vi "Begin.vi"() -> (0 "error out":errorcluster)   [LabVIEW 2013]
doc: "Called before other user functions, this VI is expected to open initial I/O refnums, load in file data, and do all program initialization. Notice that the <B>error out</B> terminal is simply used for data flow. Wiring it to other structures or subVIs ensures that this VI runs first."
uses:
  <vilib>/Rock Robotics/WPI/SafetyOutput/WPI_SafetyOutputConfigMenu.ctl
  <vilib>/Rock Robotics/WPI/DriverStation/WPI_DriverStationRobotMode2.ctl
  <vilib>/Rock Robotics/WPI/Joystick/WPI_JoystickDeviceEnum.ctl
  <vilib>/Rock Robotics/SystemInterfaces/DIO/FPGA_DIORelayChannel.ctl
  <vilib>/Rock Robotics/SystemInterfaces/DIO/FPGA_DIOChannel.ctl
  <vilib>/Rock Robotics/SystemInterfaces/Typedef/FPGA_TypedefDigitalModule.ctl
  <vilib>/Rock Robotics/WPI/Solenoid/WPI_SolenoidChannel.ctl
  TankDriveAction.ctl
  QueueAction.ctl
  <vilib>/Rock Robotics/SystemInterfaces/Typedef/FPGA_TypedefSolenoidModule.ctl
  DoubleSolenoidAction.ctl
  RollerAction.ctl
  CollectorAction.ctl
  <vilib>/Rock Robotics/SystemInterfaces/DIO/FPGA_DIOPWMChannel.ctl
  SonarAction.ctl
  <vilib>/Rock Robotics/SystemInterfaces/AI/FPGA_AIChannel.ctl
  <vilib>/Rock Robotics/SystemInterfaces/Typedef/FPGA_TypedefAnalogModule.ctl
  PressureSensorAction.ctl
  Robot Global Data.vi
  OutputErrors.vi
  <vilib>/Rock Robotics/WPI/Solenoid/WPI_SolenoidOpenSingle.vi
  <vilib>/Rock Robotics/WPI/MotorControl/WPI_MotorControlOpen Talon.vi
  <vilib>/Rock Robotics/WPI/RobotDrive/WPI_RobotDriveOpen4MotorWithTalon.vi
  <vilib>/Rock Robotics/WPI/Compressor/WPI_CompressorGetSetRefNum.vi
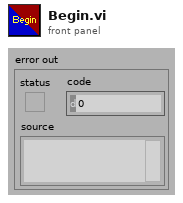
[diagram p1: front panel]
types:
  T1 = typedef "FPGA_DIOPWMChannel.ctl" = enum8{"PWM 1", "PWM 2", "PWM 3", "PWM 4", "PWM 5", "PWM 6", "PWM 7", "PWM 8", "PWM 9", "PWM 10", "Invalid"}
  T2 = typedef "PressureSensorAction.ctl" = enum16{"Init", "ReadValue", "Disable"}
  T3 = typedef "FPGA_AIChannel.ctl" = enum8{"AI 1", "AI 2", "AI 3", "AI 4", "AI 5", "AI 6", "AI 7", "AI 8", "Invalid"}
  T4 = typedef "FPGA_TypedefAnalogModule.ctl" = enum16{"Analog Module 1", "Analog Module 2"}
  T5 = typedef "SonarAction.ctl" = enum16{"Init", "ReadValue", "Disable"}
  T6 = typedef "FPGA_DIOChannel.ctl" = enum8{"DIO 1", "DIO 2", "DIO 3", "DIO 4", "DIO 5", "DIO 6", "DIO 7", "DIO 8", "DIO 9", "DIO 10", "DIO 11", "DIO 12", "DIO 13", "DIO 14", "Invalid"}
  T7 = typedef "CollectorAction.ctl" = enum16{"Init", "Raise", "Lower", "Stop", "GetStatus"}
  T8 = typedef "RollerAction.ctl" = enum16{"Init", "Off", "Forward", "Reverse"}
  T9 = typedef "FPGA_DIORelayChannel.ctl" = enum8{"Relay 1", "Relay 2", "Relay 3", "Relay 4", "Relay 5", "Relay 6", "Relay 7", "Relay 8", "Invalid"}
  T10 = typedef "FPGA_TypedefDigitalModule.ctl" = enum16{"Digital Module 1", "Digital Module 2"}
  T11 = typedef "DoubleSolenoidAction.ctl" = enum16{"Init", "Middle", "In", "Out"}
  T12 = typedef "WPI_SolenoidChannel.ctl" = enum8{"Solenoid 1", "Solenoid 2", "Solenoid 3", "Solenoid 4", "Solenoid 5", "Solenoid 6", "Solenoid 7", "Solenoid 8", "Invalid"}
  T13 = typedef "FPGA_TypedefSolenoidModule.ctl" = enum16{"Solenoid Module 1", "Solenoid Module 2"}
  T14 = typedef "QueueAction.ctl" = enum16{"Init", "SetValue", "Disable"}
  T15 = typedef "TankDriveAction.ctl" = enum16{"Init", "LinearDrive", "SetValue", "Disable"}
  T16 = typedef "WPI_JoystickDeviceEnum.ctl" = enum16{"USB 1", "USB 2", "USB 3", "USB 4", "Kinect 1", "Kinect 2"}
  T17 = typedef "WPI_DriverStationRobotMode2.ctl" = enum16{"Autonomous Disabled", "Autonomous Enabled", "Teleop Disabled", "Teleop Enabled", "Timeout", "Finish", "Test Disabled", "Test Enabled"}
  T18 = typedef "WPI_SafetyOutputConfigMenu.ctl" = enum16{"Enable", "Disable"}
  T19 = typedef "WPI_JoystickDevRef.ctl" = cluster{"Device":T16}
  T20 = typedef "WPI_RobotDriveDevRef.ctl" = cluster{"DevStatus":errorcluster, "Motors[]":T21[], "Square Inputs":bool, "Max Output":dbl, "Isochronous":bool}
  T21 = typedef "WPI_MotorControlDeviceRef.ctl" = cluster{"DeviceStatus":errorcluster, "Type":enum16{"PWM", "CAN"}, "PWM":cluster{"Digital Module":T10, "PWM Channel":T1, "DeadBand":T22}, "CAN":cluster{"Device Number":u8, "Control Mode":T23, "Semaphore":T24, "Max Vout":dbl}, "Invert":bool, "TransformRef":T25, "InvTransformRef":T25}
  T22 = typedef "WPI_PWMDeadband.ctl" = cluster{"Name":string, "maxPositivePwm":i32, "minPositivePwm":i32, "centerPwm":i32, "maxNegativePwm":i32, "minNegativePwm":i32, "angularRange":u16}
  T23 = typedef "WPI_CANJaguar_ControlMode.ctl" = enum8{"Percent VBus", "Current", "Speed", "Position", "Voltage"}
  T24 = typedef "Semaphore RefNum" = refnum<k1>
  T25 = typedef "WPI_PWMTransform_ConPane.ctl" = refnum<vi>
  T26 = typedef "WPI_CompressorDevRef.ctl" = cluster{"DevStatus":errorcluster, "DigitalInputDevRef":T27, "RelayDevRef":T28}
  T27 = typedef "WPI_DigitalInputDevRef.ctl" = cluster{"DevStatus":errorcluster, "DIO Channel":T6, "Digital Module":T10}
  T28 = typedef "WPI_RelayDevRef.ctl" = cluster{"DevStatus":errorcluster, "Relay Channel":T9, "Digital Module":T10, "Relay Direction":T29}
  T29 = typedef "WPI_RelayDirection.ctl" = enum16{"Both directions", "Forward only", "Reverse only"}
  T30 = typedef "WPI_SolenoidDevRef.ctl" = cluster{"DevStatus":errorcluster, "Solenoid Module":T13, "Forward Solenoid Channel":T12, "Reverse Solenoid Channel":T12}
  T31 = typedef "WPI_AnalogChannelDevRef.ctl" = cluster{"DevStatus":errorcluster, "Analog Module":T4, "Analog Channel":T3}
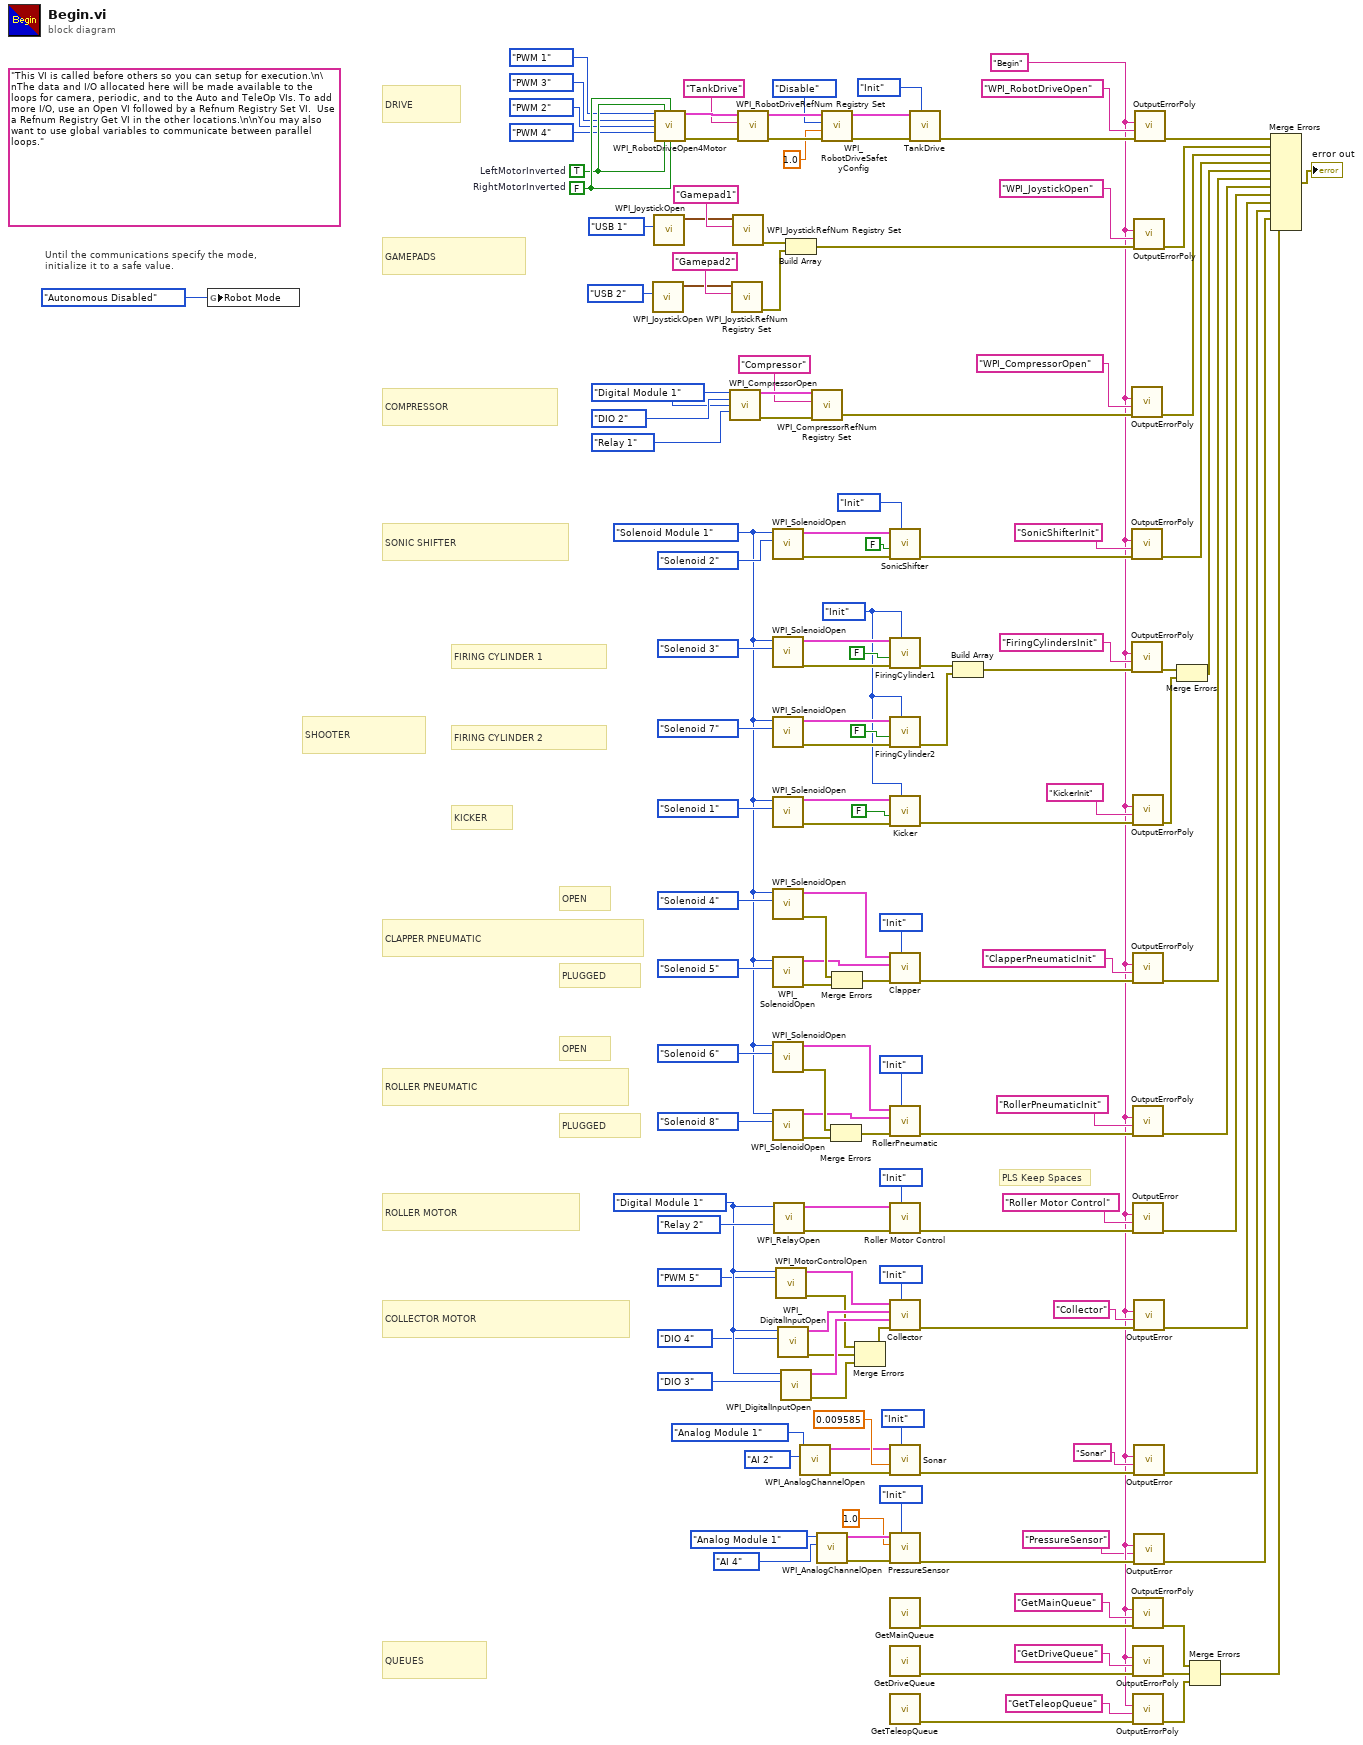
[diagram p0: block diagram]
diagram:
  w34 = FPGA_TypedefDigitalModule."Digital Module 1" ("Digital Module (Module 1)")
  w57 = FPGA_TypedefSolenoidModule."Solenoid Module 1" ("Solenoid Module (Module 1)")
  w80 = QueueAction."Init" ("Action")
  w126 = FPGA_TypedefDigitalModule."Digital Module 1" ("Pressure Switch\nand Relay Module")
  w14 = "Begin"
  (unwired) "This VI is called before others so you can setup for execution.\n\nThe data and I/O allocated here will be made available to the loops for camera, periodic, and to the Auto and TeleOp VIs. To add more I/O, use an Open VI followed by a Refnum Registry Set VI.  Use a Refnum Registry Get VI in the other locations.\n\nYou may also want to use global variables to communicate between parallel loops."
  w5 = TRUE  # LeftMotorInverted
  w6 = FALSE  # RightMotorInverted
  # "COLLECTOR MOTOR"
  # "PLS Keep Spaces"
  # "ROLLER MOTOR"
  # "PLUGGED"
  # "OPEN"
  # "PLUGGED"
  # "OPEN"
  # "ROLLER PNEUMATIC"
  # "CLAPPER PNEUMATIC"
  # "SONIC SHIFTER"
  # "QUEUES"
  # "KICKER"
  # "FIRING CYLINDER 2"
  # "FIRING CYLINDER 1"
  # "SHOOTER"
  # "COMPRESSOR"
  # "GAMEPADS"
  # "DRIVE"
  # "Until the communications specify the mode,\ninitialize it to a safe value."
  n1 = global write "Robot Global Data.vi" "Robot Mode"(WPI_DriverStationRobotMode2."Autonomous Disabled" ("Robot Mode")) -> ()
  n2 = call <vilib>:"WPI_JoystickOpen.vi"("JoystickDevice"=WPI_JoystickDeviceEnum."USB 2") -> ("JoystickDevRef"=w122:T19)  [unwired: 10 in]
  n3 = call <vilib>:"WPI_JoystickOpen.vi"("JoystickDevice"=WPI_JoystickDeviceEnum."USB 1") -> ("JoystickDevRef"=w138:T19)  [unwired: 10 in]
  n4 = call-poly <vilib>:"WPI_RobotDriveOpen4Motor.vi"("Rear Left Motor"=FPGA_DIOPWMChannel."PWM 1", "Rear Left Motor Inverted"=w5, "Rear Right Motor Inverted"=w6, "Rear Right Motor"=FPGA_DIOPWMChannel."PWM 3", "Front Left Motor"=FPGA_DIOPWMChannel."PWM 2", "Front Right Motor"=FPGA_DIOPWMChannel."PWM 4", "Front Left Motor Inverted"=w5, "Front Right Motor Inverted"=w6) -> ("RobotDriveDevRef"=w145:T20, "error out"=w143:errorcluster)  [unwired: 6 in]
  n5 = call <vilib>:"WPI_CompressorOpen.vi"("Pressure Switch Digital Module (Module 1)"=w126, "Pressure Switch DIO Channel"=FPGA_DIOChannel."DIO 2" ("Pressure Switch Channel"), "Relay Digital Module (Module 1)"=w126, "Relay Channel"=FPGA_DIORelayChannel."Relay 1") -> ("CompressorDevRef"=w130:T26, "error out"=w128:errorcluster)  [unwired: 1 in, 9 out]
  n6 = call <vilib>:"WPI_JoystickRefNum Registry Set.vi"("refnum name"="Gamepad2", "JoystickDevRef"=w122) -> ("error out"=w119:errorcluster)  [unwired: 8 in, 1 out]
  n7 = call <vilib>:"WPI_JoystickRefNum Registry Set.vi"("refnum name"="Gamepad1", "JoystickDevRef"=w138) -> ("error out"=w120:errorcluster)  [unwired: 8 in, 1 out]
  n8 = call <vilib>:"WPI_RobotDriveRefNum Registry Set.vi"("error in (no error)"=w143, "refnum name"="TankDrive", "RobotDriveDevRef"=w145) -> ("error out"=w136:errorcluster, "RobotDriveDevRef"=w142:T20)  [unwired: 7 out]
  n9 = call-poly <vilib>:"WPI_SolenoidOpen.vi"("Solenoid Channel"=WPI_SolenoidChannel."Solenoid 2", "Solenoid Module (Module 1)"=w57) -> ("error out"=w76:errorcluster, "SolenoidDevRef"=w77:T30)  [unwired: 8 in]
  n10 = call-poly <vilib>:"WPI_SolenoidOpen.vi"("Solenoid Channel"=WPI_SolenoidChannel."Solenoid 3", "Solenoid Module (Module 1)"=w57) -> ("error out"=w107:errorcluster, "SolenoidDevRef"=w110:T30)  [unwired: 8 in]
  n11 = call-poly <vilib>:"WPI_SolenoidOpen.vi"("Solenoid Channel"=WPI_SolenoidChannel."Solenoid 7", "Solenoid Module (Module 1)"=w57) -> ("error out"=w109:errorcluster, "SolenoidDevRef"=w106:T30)  [unwired: 8 in]
  n12 = call-poly <vilib>:"WPI_SolenoidOpen.vi"("Solenoid Channel"=WPI_SolenoidChannel."Solenoid 1", "Solenoid Module (Module 1)"=w57) -> ("error out"=w108:errorcluster, "SolenoidDevRef"=w105:T30)  [unwired: 8 in]
  n13 = call-poly <vilib>:"WPI_SolenoidOpen.vi"("Solenoid Channel"=WPI_SolenoidChannel."Solenoid 4", "Solenoid Module (Module 1)"=w57) -> ("error out"=w69:errorcluster, "SolenoidDevRef"=w67:T30)  [unwired: 8 in]
  n14 = call-poly <vilib>:"WPI_SolenoidOpen.vi"("Solenoid Channel"=WPI_SolenoidChannel."Solenoid 5", "Solenoid Module (Module 1)"=w57) -> ("error out"=w68:errorcluster, "SolenoidDevRef"=w65:T30)  [unwired: 8 in]
  n15 = call-poly <vilib>:"WPI_SolenoidOpen.vi"("Solenoid Channel"=WPI_SolenoidChannel."Solenoid 6", "Solenoid Module (Module 1)"=w57) -> ("error out"=w60:errorcluster, "SolenoidDevRef"=w55:T30)  [unwired: 8 in]
  n16 = call-poly <vilib>:"WPI_SolenoidOpen.vi"("Solenoid Channel"=WPI_SolenoidChannel."Solenoid 8", "Solenoid Module (Module 1)"=w57) -> ("error out"=w59:errorcluster, "SolenoidDevRef"=w54:T30)  [unwired: 8 in]
  n17 = call <vilib>:"WPI_RelayOpen.vi"("Relay Channel"=FPGA_DIORelayChannel."Relay 2", "Digital Module (Module 1)"=w34) -> ("error out"=w45:errorcluster, "RelayDevRef"=w47:T28)  [unwired: 8 in]
  n18 = call-poly <vilib>:"WPI_MotorControlOpen.vi"("PWM Channel"=FPGA_DIOPWMChannel."PWM 5", "Digital Module (Module 1)"=w34) -> ("error out"=w29:errorcluster, "MotorControlDeviceRef"=w40:T21)  [unwired: 8 in]
  n19 = call <vilib>:"WPI_DigitalInputOpen.vi"("DIO Channel"=FPGA_DIOChannel."DIO 4", "Digital Module (Module 1)"=w34) -> ("error out"=w28:errorcluster, "DigitalInputDevRef"=w36:T27)  [unwired: 8 in]
  n20 = call <vilib>:"WPI_DigitalInputOpen.vi"("DIO Channel"=FPGA_DIOChannel."DIO 3", "Digital Module (Module 1)"=w34) -> ("error out"=w27:errorcluster, "DigitalInputDevRef"=w35:T27)  [unwired: 8 in]
  n21 = Build Array(w120, w119) -> (w118:errorcluster[])
  n22 = call <vilib>:"WPI_AnalogChannelOpen.vi"("Analog Channel"=FPGA_AIChannel."AI 2", "Analog Module (Module 1)"=FPGA_TypedefAnalogModule."Analog Module 1") -> ("error out"=w19:errorcluster, "AIDeviceRef"=w18:T31)  [unwired: 8 in]
  n23 = call <vilib>:"WPI_CompressorRefNum Registry Set.vi"("error in (no error)"=w128, "refnum name"="Compressor", "CompressorDevRef"=w130) -> ("error out"=w125:errorcluster)  [unwired: 7 in, 1 out]
  n24 = call <vilib>:"WPI_AnalogChannelOpen.vi"("Analog Channel"=FPGA_AIChannel."AI 4", "Analog Module (Module 1)"=FPGA_TypedefAnalogModule."Analog Module 1") -> ("error out"=w8:errorcluster, "AIDeviceRef"=w9:T31)  [unwired: 8 in]
  n25 = call <vilib>:"WPI_RobotDriveSafetyConfig.vi"("error in (no error)"=w136, "timeout (s)"=1.0, "mode"=WPI_SafetyOutputConfigMenu."Disable", "RobotDriveDevRef"=w142) -> ("error out"=w91:errorcluster, "RobotDriveDevRef"=w92:T20)  [unwired: 6 in]
  n26 = Merge Errors(w60, w59) -> (w56:errorcluster)
  n27 = Merge Errors(w69, w68) -> (w70:errorcluster)
  n28 = Merge Errors(w29, w28, w27) -> (w30:errorcluster)
  n29 = call "SonicShifter.vi"("Action"=QueueAction."Init", "error in (no error)"=w76, "Default Position"=FALSE, "SolenoidDevRef"=w77) -> ("error out"=w74:errorcluster)  [unwired: 7 in]
  n30 = call "FiringCylinder1.vi"("Action"=w80, "error in (no error)"=w107, "Default Position"=FALSE, "SolenoidDevRef"=w110) -> ("error out"=w112:errorcluster)  [unwired: 7 in]
  n31 = call "FiringCylinder2.vi"("Action"=w80, "error in (no error)"=w109, "Default Position"=FALSE, "SolenoidDevRef"=w106) -> ("error out"=w113:errorcluster)  [unwired: 7 in]
  n32 = call "Kicker.vi"("Action"=w80, "error in (no error)"=w108, "Default Position"=FALSE, "SolenoidDevRef"=w105) -> ("error out"=w114:errorcluster)  [unwired: 7 in]
  n33 = call "Clapper.vi"("State"=DoubleSolenoidAction."Init", "Error in"=w70, "Plugged"=w65, "Open"=w67) -> ("Error out"=w63:errorcluster)  [unwired: 7 in]
  n34 = call "RollerPneumatic.vi"("State"=DoubleSolenoidAction."Init", "Error in"=w56, "Plugged"=w54, "Open"=w55) -> ("Error out"=w53:errorcluster)  [unwired: 7 in]
  n35 = call "Roller Motor Control.vi"("Action"=RollerAction."Init", "Error in"=w45, "RelayDevRef"=w47) -> ("Error out"=w44:errorcluster)  [unwired: 8 in]
  n36 = call "Collector.vi"("Action"=CollectorAction."Init", "Error in"=w30, "BottomLS"=w35, "TopLS"=w36, "Motor"=w40) -> ("Error out"=w38:errorcluster)  [unwired: 4 in, 2 out]
  n37 = call "Sonar.vi"("Action"=SonarAction."Init", "error in (no error)"=w19, "Scaling factor (V/in)"=0.009585, "AIDeviceRef"=w18) -> ("error out"=w26:errorcluster)  [unwired: 6 in, 1 out]
  n38 = call "PressureSensor.vi"("Action"=PressureSensorAction."Init", "error in (no error)"=w8, "PressureScaler"=1.0, "AIDeviceRef"=w9) -> ("error out"=w15:errorcluster)  [unwired: 6 in, 1 out]
  n39 = call "GetMainQueue.vi"() -> ("error out"=w89:errorcluster)  [unwired: 10 in, 1 out]
  n40 = call "GetDriveQueue.vi"() -> ("error out"=w88:errorcluster)  [unwired: 10 in, 1 out]
  n41 = call "GetTeleopQueue.vi"() -> ("error out"=w87:errorcluster)  [unwired: 10 in, 1 out]
  n42 = call "TankDrive.vi"("DriveAction"=TankDriveAction."Init", "error in (no error)"=w91, "RobotDriveDevRef"=w92) -> ("error out"=w90:errorcluster)  [unwired: 7 in, 1 out]
  n43 = Build Array(w112, w113) -> (w111:errorcluster[])
  n44 = call-poly "OutputErrorPoly.vi"("error in (no error)"=w125, "Causing VI"="WPI_CompressorOpen" ("Calling VI"), "Calling VI"=w14) -> ("error out"=w115:errorcluster)  [unwired: 8 in]
  n45 = call-poly "OutputErrorPoly.vi"("error in (no error)"=w74, "Causing VI"="SonicShifterInit", "Calling VI"=w14) -> ("error out"=w72:errorcluster)  [unwired: 8 in]
  n46 = call-poly "OutputErrorPoly.vi"("errors in"=w111, "Causing VI"="FiringCylindersInit", "Calling VI"=w14) -> ("error out"=w101:errorcluster)  [unwired: 8 in]
  n47 = call-poly "OutputErrorPoly.vi"("error in (no error)"=w114, "Causing VI"="KickerInit", "Calling VI"=w14) -> ("error out"=w100:errorcluster)  [unwired: 8 in]
  n48 = call-poly "OutputErrorPoly.vi"("error in (no error)"=w63, "Causing VI"="ClapperPneumaticInit", "Calling VI"=w14) -> ("error out"=w50:errorcluster)  [unwired: 8 in]
  n49 = call-poly "OutputErrorPoly.vi"("error in (no error)"=w53, "Causing VI"="RollerPneumaticInit", "Calling VI"=w14) -> ("error out"=w49:errorcluster)  [unwired: 8 in]
  n50 = call "OutputError.vi"("error in (no error)"=w44, "Causing VI"="Roller Motor Control", "Calling VI"=w14) -> ("error out"=w43:errorcluster)  [unwired: 8 in]
  n51 = call-poly "OutputErrorPoly.vi"("error in (no error)"=w89, "Causing VI"="GetMainQueue", "Calling VI"=w14) -> ("error out"=w84:errorcluster)  [unwired: 8 in]
  n52 = call-poly "OutputErrorPoly.vi"("error in (no error)"=w88, "Causing VI"="GetDriveQueue", "Calling VI"=w14) -> ("error out"=w85:errorcluster)  [unwired: 8 in]
  n53 = call-poly "OutputErrorPoly.vi"("error in (no error)"=w87, "Causing VI"="GetTeleopQueue", "Calling VI"=w14) -> ("error out"=w86:errorcluster)  [unwired: 8 in]
  n54 = call-poly "OutputErrorPoly.vi"("errors in"=w118, "Causing VI"="WPI_JoystickOpen", "Calling VI"=w14) -> ("error out"=w117:errorcluster)  [unwired: 8 in]
  n55 = call "OutputError.vi"("error in (no error)"=w38, "Causing VI"="Collector", "Calling VI"=w14) -> ("error out"=w37:errorcluster)  [unwired: 8 in]
  n56 = call "OutputError.vi"("error in (no error)"=w26, "Causing VI"="Sonar", "Calling VI"=w14) -> ("error out"=w23:errorcluster)  [unwired: 8 in]
  n57 = call "OutputError.vi"("error in (no error)"=w15, "Causing VI"="PressureSensor", "Calling VI"=w14) -> ("error out"=w16:errorcluster)  [unwired: 8 in]
  n58 = call-poly "OutputErrorPoly.vi"("error in (no error)"=w90, "Causing VI"="WPI_RobotDriveOpen", "Calling VI"=w14) -> ("error out"=w116:errorcluster)  [unwired: 8 in]
  n59 = Merge Errors(w101, w100) -> (w99:errorcluster)
  n60 = Merge Errors(w84, w85, w86) -> (w24:errorcluster)
  n61 = Merge Errors(w116, w117, w115, w72, w99, w50, w49, w43, w37, w23, w16, w24) -> (→"error out":errorcluster)
